vi "Main_PXI_Test_2.vi"() -> ()   [LabVIEW 2018]
doc: "Main VI for the controls"
uses:
  Typedefs/StateDef_Enum.ctl
  <vilib>/Utility/error.llb/DialogType.ctl
  <vilib>/Platform/TimedLoop/XDataNode/timing_clust.ctl
  <vilib>/Platform/TimedLoop/XDataNode/nitl_modes.ctl
  <vilib>/Platform/TimedLoop/XDataNode/wakeup.ctl
  <vilib>/DAQmx/read.llb/DAQmx Read (Analog 1D DBL NChan 1Samp).vi
  <vilib>/DAQmx/write.llb/DAQmx Write (Analog DBL 1Chan 1Samp).vi
  <vilib>/DAQmx/create/channels.llb/DAQmx Create Channel (AO-Voltage-Basic).vi
  <vilib>/DAQmx/create/channels.llb/DAQmx Create Channel (AI-Voltage-Basic).vi
  <vilib>/DAQmx/configure/timing.llb/DAQmx Timing (Sample Clock).vi
  <vilib>/DAQmx/create/timing.llb/DAQmx Create Timing Source (Control Loop From Task).vi
  <vilib>/DAQmx/miscellaneous.llb/DAQmx Fill In Error Info.vi
  <vilib>/Platform/TimedLoop/XDataNode/XDataNode.xnode
  Components/Timing/Timing.lvlib
  <vilib>/Platform/TimedLoop/XDataNode/XDNodeRunTimeDep.lvlib
  <resource>/objmgr/daqmx.rc
panel:
  in  "System Stop Button":bool
  in  "Pause chart?":bool
  in  "Controller Params":enum32{"Page 1"}(tab)
  in  "Kp":dbl=1.0 min=0.0
  in  "Controller On?":bool
  out "Status":string
  in  "Loop Timing":enum32{"Ctrl.", "Ref. gen", "UI"}(tab)
  in  "Ctrl.\nLoop Rate (Hz)":dbl=25000.0 format="%#_4p"
  out "# Finished\nLate counter":dbl
  in  "ConvLateErrToWarning?":bool=TRUE
  in  "UI Loop rate (Hz)":dbl=1000.0 format="%#_6p"
  in  "Display Waveforms":enum32{"Controller Signals", "DSA "}(tab)
  out "Control Effort":dbl(graph)
  out "Waveform Chart":cluster{"Double":dbl, "Numeric":dbl}(graph)
  out "DSA Signals":cluster{"Double":dbl, "Double":dbl}(graph)
  # "Control Loop Timing"
  # "Ref.  Gen. Loop Timing"
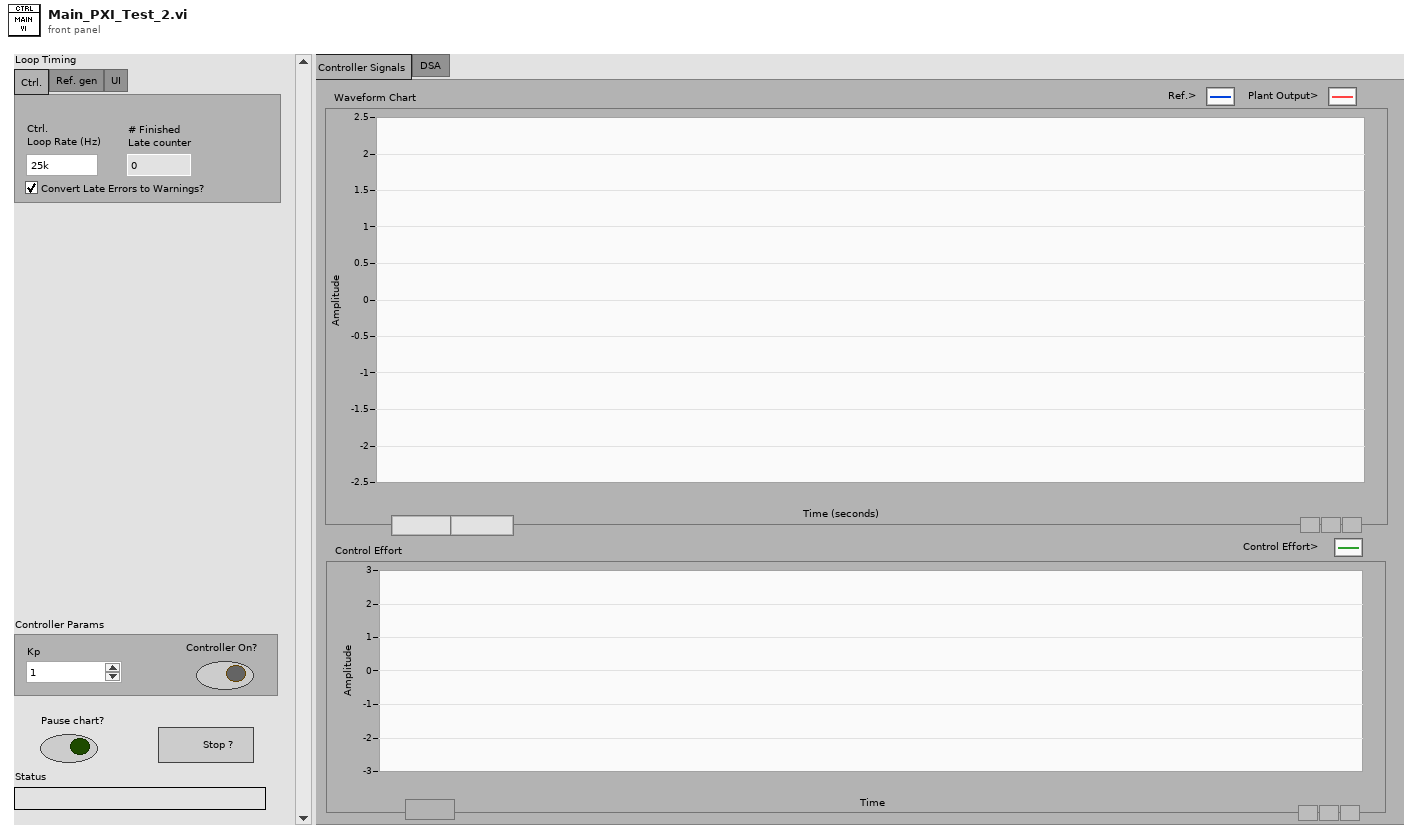
[diagram p1: front panel]
types:
  T1 = typedef "DialogType.ctl" = u16
  T2 = typedef "StateDef_Enum.ctl" = enum16{"Initialize", "Wait", "Shutdown"}
  T3 = typedef "XDNodeRunTimeDep.lvlib/timing_clust.ctl" = cluster{"Expected End [f-1]":u64, "Actual End [f-1]":u64, "Finished Late? [f-1]":bool, "Expected End [i-1]":u64, "Actual End [i-1]":u64, "Finished Late? [i-1]":bool, "Expected Start [i]":u64, "Actual Start [i]":u64, "Expected Start [f]":u64, "Actual Start [f]":u64, "Source Name":string, "Structure Name":string, "Period":i64, "Deadline":i64, "Offset":i64, "Start":i64, "Priority":i32, "Timeout":i32, "Mode":T4, "Wakeup Reason":T5, "Error":errorcluster, "Source Type":string, "Secondary Source Type":string, "Global End Time":u64, "Global Start Time":u64, "Frame Duration":u64, "Iteration Duration":u64, "Assigned CPU":i32, "I/O Scan Engine Mode":u32}
  T4 = typedef "XDNodeRunTimeDep.lvlib/nitl_modes.ctl" = enum32{"No Change", "Process missed periods, maintain original phase", "Discard missed periods, maintain original phase", "Process missed periods, ignore original phase", "Discard missed periods, ignore original phase"}
  T5 = typedef "XDNodeRunTimeDep.lvlib/wakeup.ctl" = enum32{"Normal", "Aborted", "Asynchronous wakeup", "Timing source error", "Timed loop error", "Timeout"}
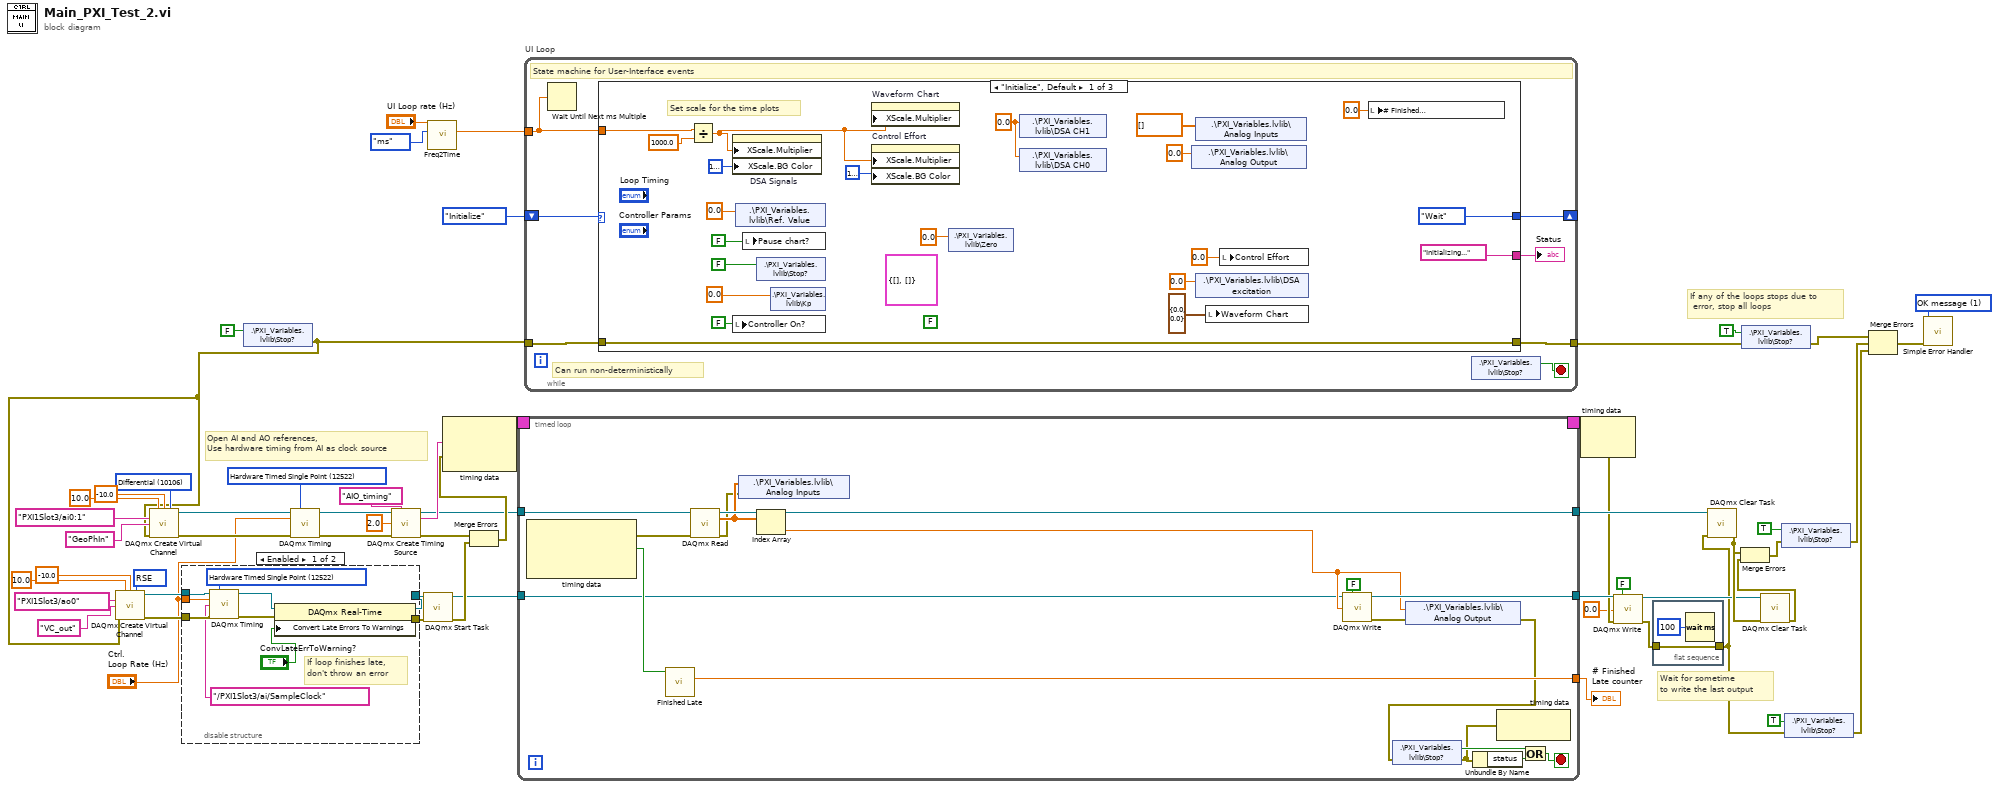
[diagram p0: block diagram]
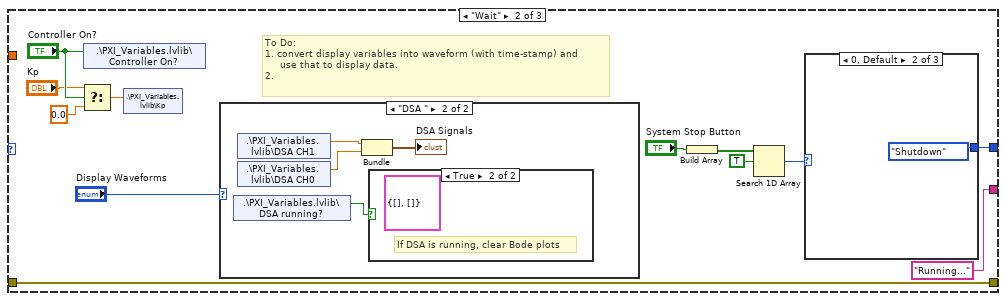
[diagram p3: hidden frame]
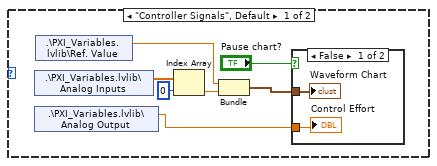
[diagram p4: hidden frame]
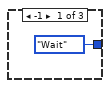
[diagram p7: hidden frame]
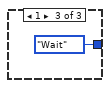
[diagram p8: hidden frame]
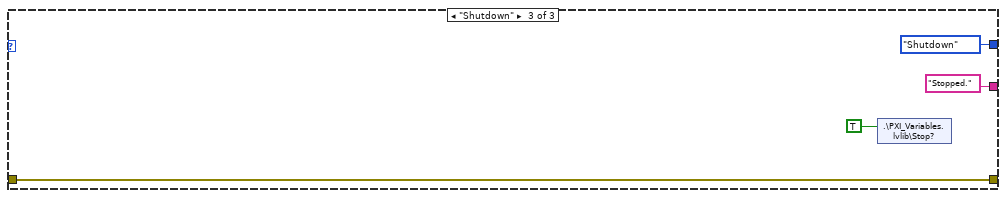
[diagram p9: hidden frame]
diagram:
  w19 = T1 1 items=["no dialog", "OK message", "continue or stop message", "OK message + warnings", "continue/stop + warnings"] ("type of dialog (OK msg:1)")
  w25 = 12522 items=["Finite Samples"=10178, "Continuous Samples"=10123, "Hardware Timed Single Point"=12522] ("sample mode")
  w41 = 10106 items=["Default"=-1, "RSE"=10083, "NRSE"=10078, "Differential"=10106, "Pseudodifferential"=12529] ("input terminal configuration")
  w44 = 10083 items=["Default"=-1, "RSE"=10083, "Differential"=10106, "Pseudodifferential"=12529] ("output terminal configuration")
  # "Wait for sometime \nto write the last output"
  # "Open AI and AO references,\nUse hardware timing from AI as clock source"
  # "If any of the loops stops due to\n error, stop all loops"
  n1 = shared-variable ".\\PXI_Variables.lvlib\\Stop?"(FALSE ("Stop?")) -> (error out=w17:errorcluster)  [unwired: 1 in]
  n2 = call-poly <vilib>:"DAQmx Create Virtual Channel.vi"("maximum value"=10.0, "minimum value"=-10.0, "output terminal configuration"=w44, "physical channels"=tag "PXI1Slot3/ao0", "name to assign"="VC_out", "error in"=w17) -> ("task out"=w9:refnum<k21>, "error out"=w8:errorcluster)  [unwired: 8 in]
  n3 = call-poly <vilib>:"DAQmx Create Virtual Channel.vi"("maximum value"=10.0, "minimum value"=-10.0, "input terminal configuration"=w41, "physical channels"=tag "PXI1Slot3/ai0:1", "name to assign"="GeoPhIn", "error in"=w17) -> ("task out"=w27:refnum<k21>, "error out"=w26:errorcluster)  [unwired: 8 in]
  n4 = disable-structure shown="Enabled" {
    disable-tunnel: w9 -> [w63 w69]
    disable-tunnel: w8 -> [w62 w68]
    disable-tunnel: "Ctrl.\nLoop Rate (Hz)" -> [w61 _]
    disable-tunnel: [w59 w68] -> w5
    disable-tunnel: [w58 w69] -> w3
    frame Enabled {
      w64 = 12522 items=["Finite Samples"=10178, "Continuous Samples"=10123, "Hardware Timed Single Point"=12522] ("sample mode")
      # "If loop finishes late,\ndon't throw an error"
      n5 = call-poly <vilib>:"DAQmx Timing.vi"("task/channels in"=w63, "sample mode"=w64, "rate"=w61, "source"=tag "/PXI1Slot3/ai/SampleClock", "error in"=w62) -> ("task out"=w66:refnum<k21>, "error out"=w65:errorcluster)  [unwired: 9 in]
      n6 = property class="DAQmx Real-Time"(reference=w66, error in=w65, "Convert Late Errors To Warnings"="ConvLateErrToWarning?") -> (reference out=w58:refnum<k21>, error out=w59:errorcluster)
    }
    frame Disabled {
    }
  }
  n7 = call-poly <vilib>:"DAQmx Timing.vi"("task/channels in"=w27, "sample mode"=w25, "rate"="Ctrl.\nLoop Rate (Hz)", "error in"=w26) -> ("task out"=w20:refnum<k21>, "error out"=w22:errorcluster)  [unwired: 10 in]
  n8 = call-poly <vilib>:"DAQmx Create Timing Source.vi"("task/channels in"=w20, "timing source name"="AIO_timing", "sleep time (us)"=2.0, "error in"=w22) -> ("task out"=w23:refnum<k21>, "timing source out"=w24:string, "error out"=w21:errorcluster)  [unwired: 9 in]
  n9 = call <vilib>:"DAQmx Start Task.vi"("task/channels in"=w3, "error in"=w5) -> ("task out"=w2:refnum<k21>, "error out"=w4:errorcluster)  [unwired: 12 in]
  n10 = call "Freq2Time.vi"("Int. Time Unit"=enum16{"sec", "us", "ms"}."ms", "Sample rate (Hz)"="UI Loop rate (Hz)") -> ("Int.  time [unit]"=w52:dbl)  [unwired: 7 in, 2 out]
  n11 = Merge Errors(w21, w4) -> (w35:errorcluster)
  n12 = node-c288(w24, w35) -> (w37:T3)
  n13 = timed-loop {
    timing: w37 -> [_]
    timing-out: [_] -> w36
    tunnel: w23 -> [w85]
    tunnel: [w83] -> w29
    tunnel: [w82] -> w28
    tunnel: w2 -> [w70]
    tunnel: [w76] -> w14
    stop <- w77 stop-if-true
    n14 = node-c288() -> (w86:errorcluster, w84:bool)  [unwired: 1 in, 1 out]
    n15 = call "Finished Late.vi"("Finished \nLate?"=w84) -> ("# Finished\nLate counter"=w83:dbl)  [unwired: 8 in, 2 out]
    n16 = call-poly <vilib>:"DAQmx Read.vi"("task/channels in"=w85, "error in"=w86) -> ("task out"=w82:refnum<k21>, "data"=w81:dbl[], "error out"=w75:errorcluster)  [unwired: 11 in]
    n17 = shared-variable ".\\PXI_Variables.lvlib\\Analog Inputs"(w81, error in=w75) -> ()  [unwired: 1 out]
    n18 = Index Array(array=w81) -> (element=w71:dbl)  [unwired: 1 in]
    n19 = call-poly <vilib>:"DAQmx Write.vi"("task/channels in"=w70, "auto start"=FALSE, "data"=w71) -> ("task out"=w76:refnum<k21>, "error out"=w74:errorcluster)  [unwired: 10 in, 1 out]
    n20 = shared-variable ".\\PXI_Variables.lvlib\\Analog Output"(w71, error in=w74) -> (error out=w73:errorcluster)
    n21 = shared-variable ".\\PXI_Variables.lvlib\\Stop?"(error in=w73) -> (w80:bool, error out=w79:errorcluster)
    n22 = Unbundle By Name(w79) -> ("status"=w78:bool)
    n23 = node-c288(w79) -> ()  [unwired: 1 out]
    n24 = Or(x=w80, y=w78) -> (x .or. y?=w77:bool)
  }
  "# Finished\nLate counter" <- w29
  n25 = while "UI Loop" {
    shift-right: [w98] -> _
    shift-left: StateDef_Enum."Initialize" ("State defining Enum") -> [w99]
    tunnel: w17 -> [w97]
    tunnel: [w96] -> w51
    tunnel: w52 -> [w93]
    stop <- w94 stop-if-true
    # "Can run non-deterministically"
    # "State machine for User-Interface events"
    n26 = Wait Until Next ms Multiple(millisecond multiple=w93) -> ()  [unwired: 1 out]
    n27 = case shown="\"Initialize\", Default" w99 {
      tunnel: [StateDef_Enum."Wait" ("State defining Enum") w129 StateDef_Enum."Shutdown" ("State defining Enum")] -> w98
      tunnel: w97 -> [w117 w127 w152]
      tunnel: [w117 w127 w152] -> w96
      tunnel: ["Initializing..." ("Status") "Running..." ("Status") "Stopped." ("Status")] -> w95
      tunnel: w93 -> [w115 _ _]
      frame "Initialize", Default {
        w101 = 0.0 ("DSA CH1")
        (unwired) cluster{dbl[], dbl[]} {[], []} ("Magnitude Bode Plot")
        (unwired) FALSE ("DSA \nRunning?")
        # "Set scale for the time plots"
        n28 = Divide(x=w115, y=1000.0) -> (x/y=w109:dbl)
        n29 = property on="DSA Signals" class="WFChart (strict)"("XScale.Multiplier"=w109, "XScale.BG Color"=u32 16777216) -> ()  [unwired: 2 in, 2 out]
        n30 = local write "Controller On?"(FALSE ("Controller On?")) -> ()
        n31 = shared-variable ".\\PXI_Variables.lvlib\\Ref. Value"(0.0 ("Ref. Value")) -> ()  [unwired: 1 in, 1 out]
        n32 = local write "Pause chart?"(FALSE ("Pause chart?")) -> ()
        n33 = shared-variable ".\\PXI_Variables.lvlib\\Stop?"(FALSE ("Stop?")) -> ()  [unwired: 1 in, 1 out]
        n34 = shared-variable ".\\PXI_Variables.lvlib\\Kp"(0.0 ("Kp")) -> ()  [unwired: 1 in, 1 out]
        n35 = property on="Waveform Chart" class="WFChart (strict)"("XScale.Multiplier"=w109) -> ()  [unwired: 2 in, 2 out]
        n36 = property on="Control Effort" class="WFChart (strict)"("XScale.Multiplier"=w109, "XScale.BG Color"=u32 16777216) -> ()  [unwired: 2 in, 2 out]
        n37 = shared-variable ".\\PXI_Variables.lvlib\\Zero"(0.0 ("Zero")) -> ()  [unwired: 1 in, 1 out]
        n38 = shared-variable ".\\PXI_Variables.lvlib\\DSA CH1"(w101) -> ()  [unwired: 1 in, 1 out]
        n39 = shared-variable ".\\PXI_Variables.lvlib\\DSA CH0"(w101) -> ()  [unwired: 1 in, 1 out]
        n40 = shared-variable ".\\PXI_Variables.lvlib\\Analog Output"(0.0 ("Analog Output")) -> ()  [unwired: 1 in, 1 out]
        n41 = shared-variable ".\\PXI_Variables.lvlib\\Analog Inputs"(dbl[] [] ("Analog Inputs")) -> ()  [unwired: 1 in, 1 out]
        n42 = shared-variable ".\\PXI_Variables.lvlib\\DSA excitation"(0.0 ("DSA excitation")) -> ()  [unwired: 1 in, 1 out]
        n43 = local write "Waveform Chart"(cluster{"Double":dbl, "Numeric":dbl} {"Double"=0.0, "Numeric"=0.0} ("Waveform Chart")) -> ()
        n44 = local write "Control Effort"(0.0 ("Control Effort")) -> ()
        n45 = local write "# Finished\nLate counter"(0.0 ("# Finished\nLate counter")) -> ()
      }
      frame "Wait" {
        # "To Do:\n1. convert display variables into waveform (with time-stamp) and\n     use that to display data.\n2."
        n46 = Select(t="Kp", s="Controller On?", f=0.0) -> (s? t:f=w125:dbl)
        n47 = shared-variable ".\\PXI_Variables.lvlib\\Controller On?"("Controller On?") -> ()  [unwired: 1 in, 1 out]
        n48 = shared-variable ".\\PXI_Variables.lvlib\\Kp"(w125) -> ()  [unwired: 1 in, 1 out]
        n49 = case shown="\"DSA \"" "Display Waveforms" {
          frame "Controller Signals", Default {
            n50 = shared-variable ".\\PXI_Variables.lvlib\\Analog Inputs"() -> (w139:dbl[])  [unwired: 1 in, 1 out]
            n51 = shared-variable ".\\PXI_Variables.lvlib\\Analog Output"() -> (w133:dbl)  [unwired: 1 in, 1 out]
            n52 = shared-variable ".\\PXI_Variables.lvlib\\Ref. Value"() -> (w136:dbl)  [unwired: 1 in, 1 out]
            n53 = Index Array(array=w139, index=0) -> (element=w138:dbl)
            n54 = Bundle("Double"=w136, "Numeric"=w138) -> (w134:cluster{"Double":dbl, "Numeric":dbl})  [unwired: 1 in]
            n55 = case shown="False" "Pause chart?" {
              tunnel: w134 -> [w141 _]
              tunnel: w133 -> [w140 _]
              frame False {
                "Waveform Chart" <- w141
                "Control Effort" <- w140
              }
              frame True {
              }
            }
          }
          frame "DSA " {
            n56 = shared-variable ".\\PXI_Variables.lvlib\\DSA running?"() -> (w142:bool)  [unwired: 1 in, 1 out]
            n57 = shared-variable ".\\PXI_Variables.lvlib\\DSA CH1"() -> (w144:dbl)  [unwired: 1 in, 1 out]
            n58 = shared-variable ".\\PXI_Variables.lvlib\\DSA CH0"() -> (w143:dbl)  [unwired: 1 in, 1 out]
            n59 = Bundle("Double"=w144, "Double"=w143) -> (→"DSA Signals":cluster{"Double":dbl, "Double":dbl})  [unwired: 1 in]
            n60 = case shown="True" w142 {
              frame False {
              }
              frame True {
                (unwired) cluster{dbl[], dbl[]} {[], []} ("Magnitude Bode Plot")
                # "If DSA is running, clear Bode plots"
              }
            }
          }
        }
        n61 = Build Array("System Stop Button") -> (w131:bool[])
        n62 = Search 1D Array(1D array=w131, element=TRUE) -> (index of element=w128:i32)  [unwired: 1 in]
        n63 = case shown="0, Default" w128 {
          tunnel: [StateDef_Enum."Wait" ("State defining Enum") StateDef_Enum."Shutdown" ("State defining Enum") StateDef_Enum."Wait" ("State defining Enum")] -> w129
          frame -1 {
          }
          frame 0, Default {
          }
          frame 1 {
          }
        }
      }
      frame "Shutdown" {
        n64 = shared-variable ".\\PXI_Variables.lvlib\\Stop?"(TRUE) -> ()  [unwired: 1 in, 1 out]
      }
    }
    "Status" <- w95
    n65 = shared-variable ".\\PXI_Variables.lvlib\\Stop?"() -> (w94:bool)  [unwired: 1 in, 1 out]
  }
  n66 = node-c288(w36) -> (w13:errorcluster)
  n67 = call-poly <vilib>:"DAQmx Write.vi"("task/channels in"=w14, "auto start"=FALSE, "data"=0.0, "error in"=w13) -> ("task out"=w10:refnum<k21>, "error out"=w11:errorcluster)  [unwired: 9 in, 1 out]
  n68 = flat-sequence {
    tunnel: [w154] -> w1
    tunnel: w11 -> [w154]
    frame #0 {
      n69 = Wait (ms)(milliseconds to wait=u32 100) -> ()  [unwired: 1 out]
    }
  }
  n70 = call <vilib>:"DAQmx Clear Task.vi"("task in"=w28, "error in"=w1) -> ("error out"=w15:errorcluster)  [unwired: 13 in]
  n71 = shared-variable ".\\PXI_Variables.lvlib\\Stop?"(TRUE ("Stop?"), error in=w51) -> (error out=w50:errorcluster)
  n72 = call <vilib>:"DAQmx Clear Task.vi"("task in"=w10, "error in"=w15) -> ("error out"=w32:errorcluster)  [unwired: 13 in]
  n73 = Merge Errors(w15, w32) -> (w33:errorcluster)
  n74 = shared-variable ".\\PXI_Variables.lvlib\\Stop?"(TRUE ("Stop?"), error in=w33) -> (error out=w30:errorcluster)
  n75 = shared-variable ".\\PXI_Variables.lvlib\\Stop?"(TRUE ("Stop?"), error in=w1) -> (error out=w31:errorcluster)
  n76 = Merge Errors(w50, w30, w31) -> (w56:errorcluster)
  n77 = call <vilib>:"Simple Error Handler.vi"("type of dialog (OK msg:1)"=w19, "error in (no error)"=w56) -> ()  [unwired: 3 in, 5 out]
